vi "Configure Export Signal.vi"(8 "error in (no error)":errorcluster, 11 "FGen PXI Base CFG in":refnum<class "Generate DC CFG.lvclass">) -> (0 "error out":errorcluster, 3 "FGen PXI Base CFG out":refnum<class "Generate DC CFG.lvclass">)   [LabVIEW 2023, in "FGen Simulated CFGs.lvlib" / "Generate DC CFG.lvclass"]
uses:
  Generate DC CFG.lvclass
  83dfbe61-3606-4481-8714-31fd42503d22.vi
  <vilib>/Utility/error.llb/Error Cluster From Error Code.vi
  <vilib>/ErrorRing/Error Ring.xnode
  Configuration/Configuration JSON/Configuration JSON Base/CFG JSON.lvclass
  D:/git/HAL/HAL GOOP4/Configuration JSON Base/CFG JSON.lvclass
  D:/git/HAL/HAL GOOP4/Interfaces/IConfigure/IConfigure.lvclass
  D:/git/HAL/HAL GOOP4/FGen/FGen Simulated/Configurations/Generate DC CFG/Generate DC CFG.lvclass
panel:
  out "Data":T1
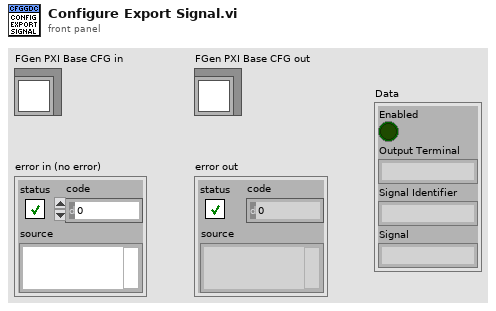
[diagram p1: front panel]
types:
  T1 = cluster{"Enabled":bool, "Output Terminal":string, "Signal Identifier":string, "Signal":string}
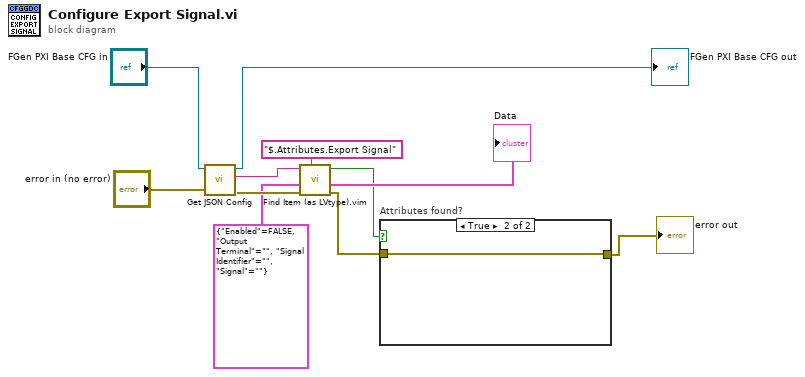
[diagram p0: block diagram]
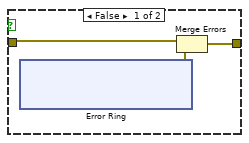
[diagram p2: hidden frame]
diagram:
  n1 = call "Get JSON Config.vi"("error in (no error)"="error in (no error)", "CFG Base in"="FGen PXI Base CFG in") -> ("error out"=w7:errorcluster, "<JSON>Config>"=w5:string, "CFG Base out"=→"FGen PXI Base CFG out":refnum<class "Generate DC CFG.lvclass">)  [unwired: 7 in]
  n2 = call "Find Item (as LVtype).vim"("$Path or Item Name"="$.Attributes.Export Signal", "error in (no error)"=w7, "Data Type and Default Value"=T1 {"Enabled"=FALSE, "Output Terminal"="", "Signal Identifier"="", "Signal"=""}, "JSON"=w5) -> ("error out"=w3:errorcluster, "Data"=→"Data":T1, "Found"=w2:bool)  [unwired: 4 in, 1 out]
  n3 = case "Attributes found?" shown="True" w2 {
    tunnel: [w14 w20] -> w1
    tunnel: w3 -> [w13 w20]
    frame False {
      n4 = xnode "Error Ring"() -> ("error out"=w12:errorcluster)
      n5 = Merge Errors(w13, w12) -> (w14:errorcluster)
    }
    frame True {
    }
  }
  "error out" <- w1
